vi "PID_test.vi"() -> ()   [LabVIEW 2015]
uses:
  BERTTA.dll
panel:
  out "last_timeChange":dbl
  out "Waveform Chart":dynamicdata(graph)
  out "Tr":dbl
  out "seconds":dbl
  out "lastErr":dbl
  out "errSum":dbl
  out "output":dbl
  in  "port":i32=9
  in  "kd":dbl
  in  "ki":dbl=1.0
  in  "kp":dbl=5.0
  in  "Setpoint":dbl
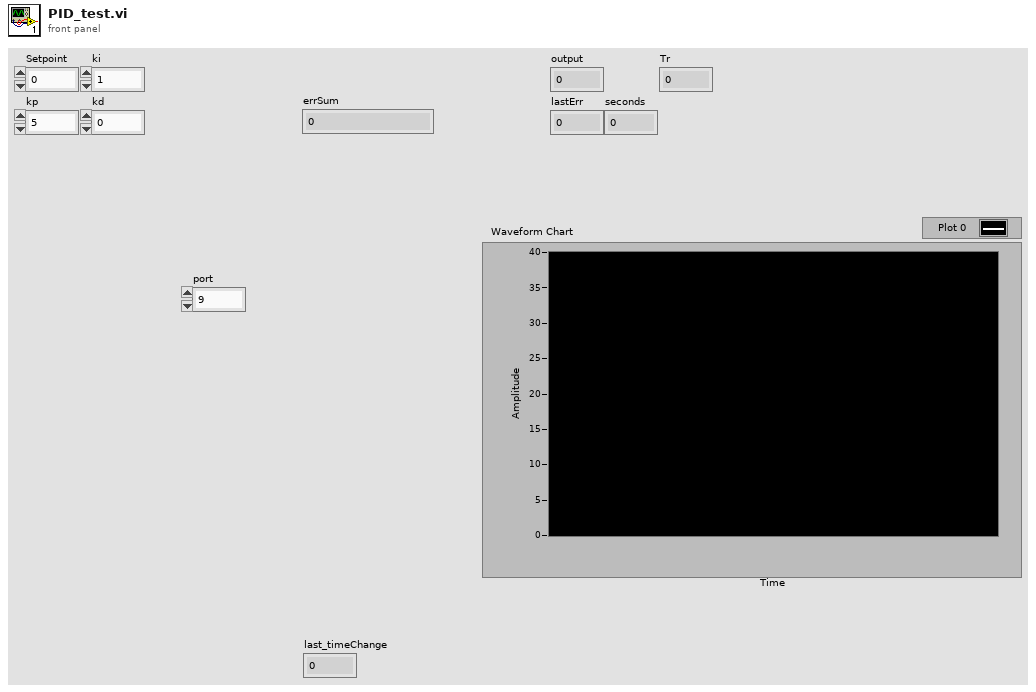
[diagram p1: front panel]
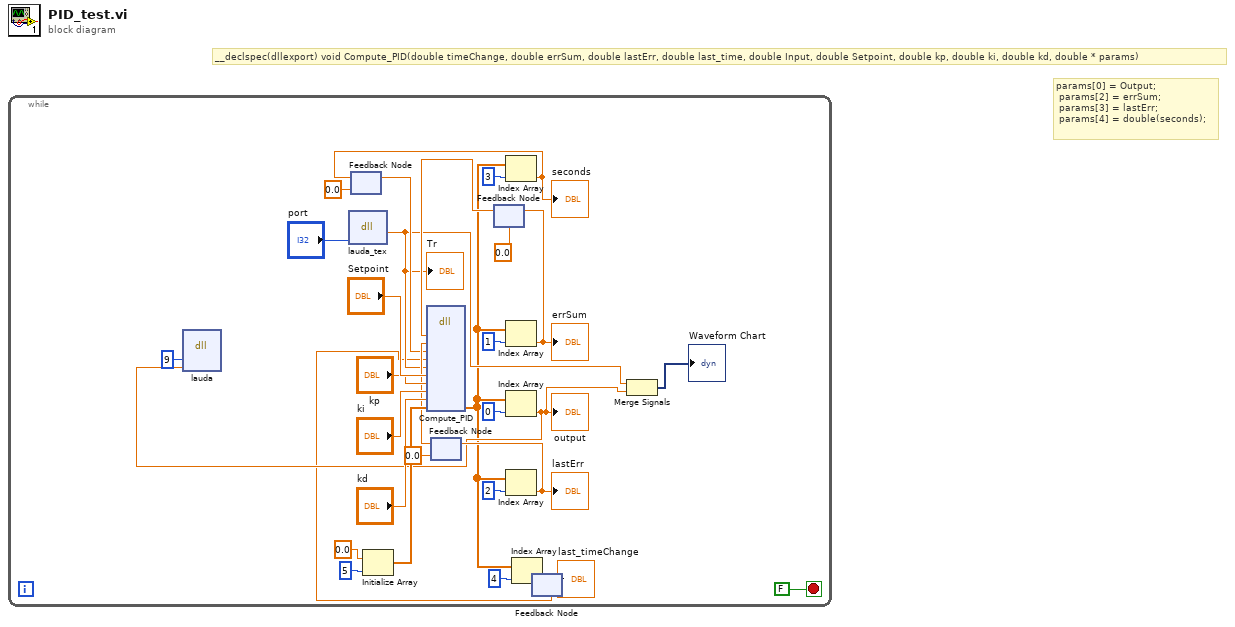
[diagram p0: block diagram]
diagram:
  # "params[0] = Output;\n\tparams[2] = errSum;\n\tparams[3] = lastErr;\n\tparams[4] = double(seconds);"
  # "__declspec(dllexport) void Compute_PID(double timeChange, double errSum, double lastErr, double last_time, double Input, double Setpoint, double kp, double ki, double kd, double * params)"
  n1 = while {
    stop <- FALSE stop-if-true
    n2 = dll-call lib="C:/Users/shresplab/OneDrive - Kemira Oyj/Documents/Visual Studio 2017/Projects/Bertta/BERTTA/x64/Debug/BERTTA.dll" fn="lauda_tex"("port"="port") -> ("return type"=w9:dbl)  [unwired: 4 in, 2 out]
    "Tr" <- w9
    n3 = feedback #1(0.0) -> (w14:dbl)
    n4 = Initialize Array(0.0 ("element"), 5 ("dimension size")) -> (w24:dbl[])
    n5 = feedback #2(0.0) -> (w16:dbl)
    n6 = feedback #3(0.0) -> (w18:dbl)
    n7 = feedback #4() -> (w1:dbl)  [unwired: 1 in]
    "last_timeChange" <- w1
    n8 = dll-call lib="C:/Users/shresplab/OneDrive - Kemira Oyj/Documents/Visual Studio 2017/Projects/Bertta/BERTTA/x64/Debug/BERTTA.dll" fn="Compute_PID"("errSum"=w18, "lastErr"=w16, "last_time"=w14, "last_timeChange"=w1, "Input"=w9, "Setpoint"="Setpoint", "kp"="kp", "ki"="ki", "kd"="kd", "params"=w24) -> ("params"=w3:dbl[])  [unwired: 13 in, 2 out]
    n9 = Index Array(array=w3, index=3) -> (element=w15:dbl)
    "seconds" <- w15
    n10 = feedback-in #1(w15) -> ()
    n11 = Index Array(array=w3, index=1) -> (element=w19:dbl)
    "errSum" <- w19
    n12 = feedback-in #3(w19) -> ()
    n13 = Index Array(array=w3, index=0) -> (element=w8:dbl)
    "output" <- w8
    n14 = dll-call lib="C:/Users/shresplab/OneDrive - Kemira Oyj/Documents/Visual Studio 2017/Projects/Bertta/BERTTA/x64/Debug/BERTTA.dll" fn="lauda"("port"=9, "set_temp"=w8) -> ()  [unwired: 6 in, 2 out]
    n15 = Index Array(array=w3, index=2) -> (element=w17:dbl)
    "lastErr" <- w17
    n16 = feedback-in #2(w17) -> ()
    n17 = Index Array(array=w3, index=4) -> (element=w2:dbl)
    n18 = feedback-in #4(w2) -> ()
    n19 = Merge Signals(w9, w8) -> (→"Waveform Chart":dynamicdata)
  }
